vi "Stop.vi"(8 "error in (no error)":errorcluster, 10 "Message in":refnum<class "StopMessage.lvclass">, 11 "Waveform in":refnum<class "Waveform.lvclass">) -> (0 "error out":errorcluster, 3 "Waveform out":refnum<class "Waveform.lvclass">)   [LabVIEW 2012, in "Waveform.lvclass"]
doc: "This member function is called when the statemachine in the run.vi receives an 'stop' command. It relays the message to all observers of the component.\n\nOverride this member function in your derived class if you need additional stop functionality (but don't forget to call the parent method)."
uses:
  Waveform.lvclass
  <vilib>/Distrio/Murmex/StopMessage/StopMessage.lvclass
  <vilib>/Distrio/Murmex/Murmex/Murmex.lvclass
  Waveform.lvclass/Waveform.ctl
panel:
  # "This method is called when the STOP\ntrigger is sent. \n\nOverride this method when your component needs to\nrespond to this trigger. \n\nCall parent for proper implementation"
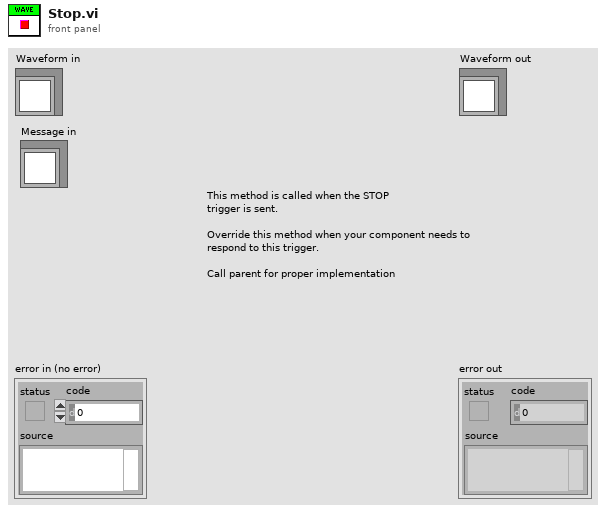
[diagram p1: front panel]
types:
  T1 = enum8{"Enabled", "Disabled", "Disabled and Grayed Out"}
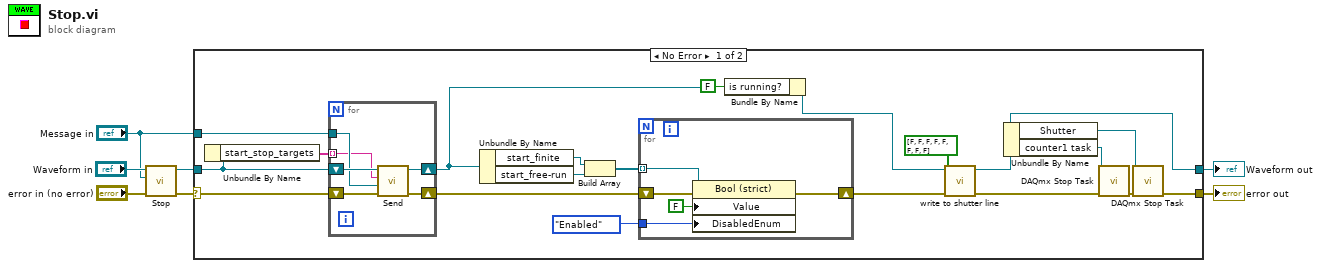
[diagram p0: block diagram]
diagram:
  n1 = call-parent "Stop.vi"("error in (no error)"="error in (no error)", "Message in"="Message in", "Murmex in"="Waveform in") -> ("error out"=w5:errorcluster, "Murmex out"=w4:refnum<class "Waveform.lvclass">)  [unwired: 7 in]
  n2 = case shown="No Error" w5 {
    selector: w5 -> [w22 w39]
    tunnel: w4 -> [w18 w40]
    tunnel: [w9 w40] -> w3
    tunnel: [w14 w39] -> w2
    tunnel: "Message in" -> [w19 _]
    frame No Error {
      n3 = Unbundle By Name(w18) -> ("start_stop_targets"=w17:string[])
      n4 = for {
        shift-right: [w30] -> w21
        shift-left: w22 -> [w31]
        shift-right: [w32] -> w20
        shift-left: w18 -> [w33]
        tunnel: w19 -> [w29]
        tunnel: w17 -> [w28] mode=indexing
        n5 = call <vilib>:"Send.vi"("error in (no error)"=w31, "Message"=w29, "recipient"=w28, "Murmex in"=w33) -> ("error out"=w30:errorcluster, "Murmex out"=w32:refnum<class "Waveform.lvclass">)  [unwired: 6 in]
      }
      n6 = Unbundle By Name(w20) -> ("start_finite"=w26:refnum<vi>, "start_free-run"=w27:refnum<vi>)
      n7 = Build Array(w26, w27) -> (w25:refnum<vi>[])
      n8 = for {
        tunnel: w25 -> [w37] mode=indexing
        shift-right: [w34] -> w12
        shift-left: w21 -> [w38]
        tunnel: T1."Enabled" ("Disabled") -> [w35]
        n9 = property class="Bool (strict)"(reference=w37, error in=w38, "Value"=FALSE, "DisabledEnum"=w35) -> (error out=w34:errorcluster)  [unwired: 1 out]
      }
      n10 = Bundle By Name(cluster=w20, "is running?"=FALSE ("runtime.is running?")) -> (w10:refnum<class "Waveform.lvclass">)
      n11 = call-dynamic "write to shutter line.vi"("error in (no error)"=w12, "Output Array"=bool[] [FALSE, FALSE, FALSE, FALSE, FALSE, FALSE, FALSE, FALSE], "Waveform in"=w10) -> ("error out"=w11:errorcluster, "Waveform out"=w9:refnum<class "Waveform.lvclass">)  [unwired: 7 in]
      n12 = Unbundle By Name(w9) -> ("Shutter"=w13:refnum<k21>, "counter1 task"=w16:refnum<k21>)
      n13 = call <vilib>:"DAQmx Stop Task.vi"("task/channels in"=w16, "error in"=w11) -> ("error out"=w15:errorcluster)  [unwired: 12 in, 1 out]
      n14 = call <vilib>:"DAQmx Stop Task.vi"("task/channels in"=w13, "error in"=w15) -> ("error out"=w14:errorcluster)  [unwired: 12 in, 1 out]
    }
    frame Error {
    }
  }
  "error out" <- w2
  "Waveform out" <- w3
